vi "write_DAC.vi"() -> ()   [LabVIEW 2014]
uses:
  aardvark.dll
panel:
  out "Dup Aardvark Handle":i32
  out "DAC Written":bool
  out "error out":errorcluster
  in  "DAC_ADD":u16[](array[numeric]) format="%.0x"
  in  "DAC_Val":u16 format="%.0x"
  in  "error in (no error)":errorcluster
  in  "Address (0x50) in":u16=80 max=1023 format="%.0x"
  in  "Aardvark Handle in":i32 min=0
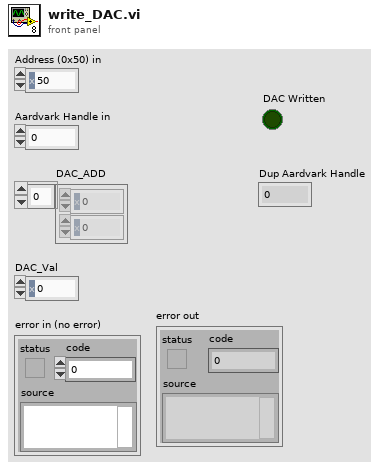
[diagram p1: front panel]
types:
  T1 = cluster{"unsigned byte array[0]":u8, "unsigned byte array[1]":u8, "unsigned byte array[2]":u8, "unsigned byte array[3]":u8, "unsigned byte array[4]":u8, "unsigned byte array[5]":u8, "unsigned byte array[6]":u8, "unsigned byte array[7]":u8, "unsigned byte array[8]":u8}
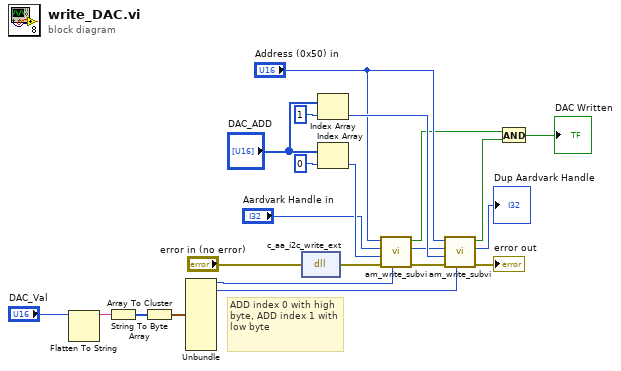
[diagram p0: block diagram]
diagram:
  # "ADD index 0 with high byte, ADD index 1 with low byte"
  n1 = Flatten To String(anything="DAC_Val") -> (data string=w15:string)  [unwired: 3 in, 2 out]
  n2 = String To Byte Array(string=w15) -> (unsigned byte array=w16:u8[])
  n3 = Array To Cluster(array=w16) -> (cluster=w17:T1)
  n4 = Unbundle(w17) -> ("unsigned byte array[0]"=w11:u8, "unsigned byte array[1]"=w10:u8)  [unwired: 7 out]
  n5 = dll-call lib="aardvark.dll" fn="c_aa_i2c_write_ext"(error in="error in (no error)") -> (error out=w14:errorcluster)  [unwired: 3 in, 1 out]
  n6 = Index Array(array="DAC_ADD", index=1) -> (element=w8:u16)
  n7 = Index Array(array="DAC_ADD", index=0) -> (element=w9:u16)
  n8 = call "am_write_subvi.vi"("Data to Write"=w11, "error in (no error)"=w14, "Memory ADD"=w9, "Aardvark Handle in"="Aardvark Handle in", "Address (0x50) in"="Address (0x50) in") -> ("error out"=w13:errorcluster, "Dup Aardvark Handle"=w5:i32, "Data Written"=w4:bool)  [unwired: 4 in]
  n9 = call "am_write_subvi.vi"("Data to Write"=w10, "error in (no error)"=w13, "Memory ADD"=w8, "Aardvark Handle in"=w5, "Address (0x50) in"="Address (0x50) in") -> ("error out"=→"error out":errorcluster, "Dup Aardvark Handle"=→"Dup Aardvark Handle":i32, "Data Written"=w3:bool)  [unwired: 4 in]
  n10 = And(x=w4, y=w3) -> (x .and. y?=→"DAC Written":bool)
